vi "VI Server_GetControlClassNameAndType.vi"(7 "Label":string, 8 "error in (no error)":errorcluster, 11 "VI Server Cluster":T2) -> (0 "error out":errorcluster, 1 "ClassName":string, 2 "ControlType":T1, 3 "VI Server Cluster.DUP":T2)   [LabVIEW 2020, in "VI Server Toolkit LV2013.lvlib"]
doc: "Returns control class name and its type (digital, Boolean, etc.)\nRequires control's label input."
uses:
  VI Server Toolkit LV2013.lvlib
  VI Server_TypeDefs/VI Server_RefsCluster.ctl
  VI Server_TypeDefs/VI Server_DataType.ctl
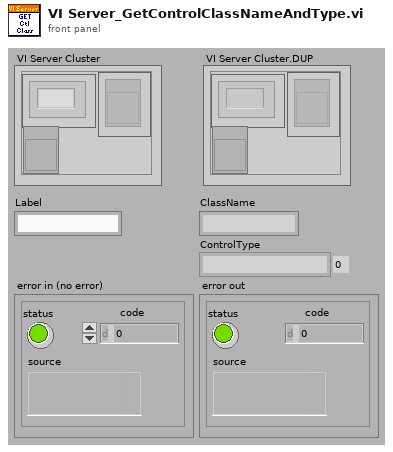
[diagram p1: front panel]
types:
  T1 = typedef "VI Server Toolkit LV2013.lvlib/VI Server_DataType.ctl" = enum16{"", "Digital [Dbl]", "Digital [Sgl]", "Digital [I32]", "Digital [I16]", "Digital [I8]", "Digital [U32]", "Digital [U16]", "Digital [U8]", "Boolean", "Slide [Dbl]", "Slide [Sgl]", "Slide [I32]", "Slide [I16]", "Slide [I8]", "Slide [U32]", "Slide [U16]", "Slide [U8]", "Enumerated", "Path", "VISA Resource Name", "Text Ring", "String", "TabControl", "Knob [U8]", "Knob [U16]", "Knob [U32]", "Knob [I8]", "Knob [I16]", "Knob [I32]", "Knob [SGL]", "Knob [DBL]"}
  T2 = typedef "VI Server_RefsCluster.ctl" = cluster{"Labels":string[], "Refs":refnum<vi>[], "VI Ref":refnum<vi>}
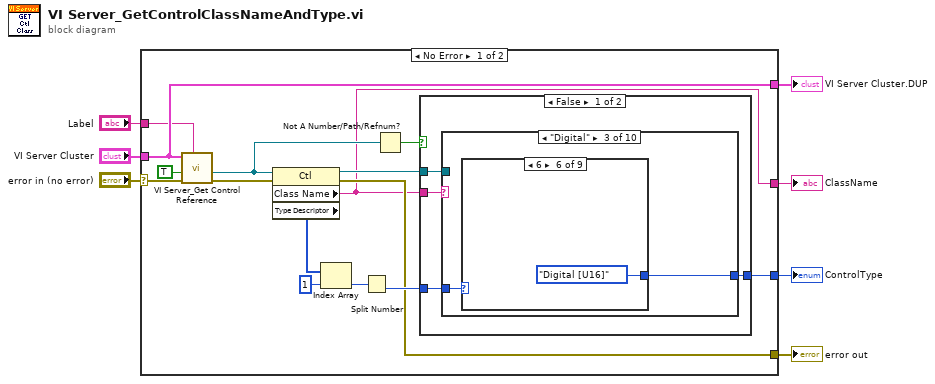
[diagram p0: block diagram]
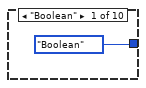
[diagram p2: hidden frame]
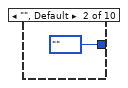
[diagram p3: hidden frame]
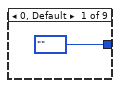
[diagram p4: hidden frame]
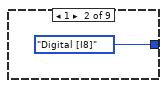
[diagram p5: hidden frame]
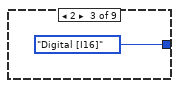
[diagram p6: hidden frame]
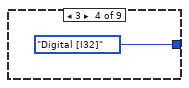
[diagram p7: hidden frame]
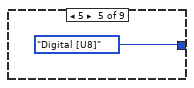
[diagram p8: hidden frame]
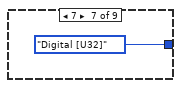
[diagram p9: hidden frame]
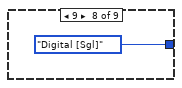
[diagram p10: hidden frame]
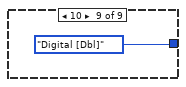
[diagram p11: hidden frame]
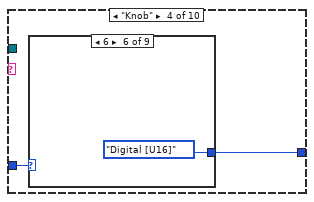
[diagram p12: hidden frame]
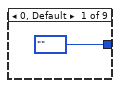
[diagram p13: hidden frame]
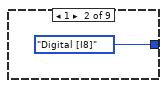
[diagram p14: hidden frame]
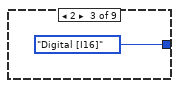
[diagram p15: hidden frame]
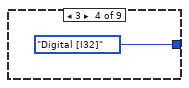
[diagram p16: hidden frame]
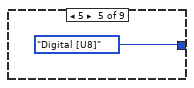
[diagram p17: hidden frame]
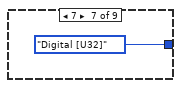
[diagram p18: hidden frame]
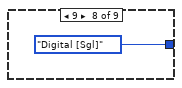
[diagram p19: hidden frame]
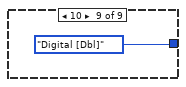
[diagram p20: hidden frame]
diagram:
  n1 = case shown="No Error" "error in (no error)" {
    selector: "error in (no error)" -> [w17 w69]
    tunnel: [w10 w69] -> w7
    tunnel: "VI Server Cluster" -> [w15 _]
    tunnel: "Label" -> [w14 _]
    tunnel: [w15 _] -> w3
    tunnel: [w11 VI_Server_DataType."" ("ControlType 2")] -> w2
    tunnel: [w9 _] -> w1
    frame No Error {
      n2 = call "VI Server_Get Control Reference.vi"("Label"=w14, "error in"=w17, "Single Instance (T)"=TRUE, "VI Server Cluster"=w15) -> ("error out"=w16:errorcluster, "Control Reference (Generic)"=w13:refnum<vi>)  [unwired: 4 in, 2 out]
      n3 = property class="Ctl"(reference=w13, error in=w16) -> (reference out=w18:refnum<vi>, error out=w10:errorcluster, "Class Name"=w9:string, "Type Descriptor"=w20:i16[])
      n4 = Index Array(array=w20, index=1) -> (element=w21:i16)
      n5 = Split Number(x=w21) -> (lo(x)=w19:u8)  [unwired: 1 out]
      n6 = Not A Number/Path/Refnum?(number/path/refnum=w13) -> (NaN/Path/Refnum?=w12:bool)
      n7 = case shown="False" w12 {
        tunnel: w9 -> [w26 _]
        tunnel: w19 -> [w25 _]
        tunnel: w18 -> [w24 _]
        tunnel: [w23 VI_Server_DataType."" ("ControlType 2")] -> w11
        frame False {
          n8 = case shown="\"Digital\"" w26 {
            tunnel: w25 -> [_ _ w30 w41 w52 _ _ _ _ _]
            tunnel: w24 -> [_ _ _ _ _ _ _ _ _ _]
            tunnel: [VI_Server_DataType."Boolean" ("ControlType 2") VI_Server_DataType."" ("ControlType 2") w29 w40 w51 VI_Server_DataType."Enumerated" ("ControlType 2") VI_Server_DataType."Path" ("ControlType 2") VI_Server_DataType."VISA Resource Name" ("ControlType 2") VI_Server_DataType."Text Ring" ("ControlType 2") VI_Server_DataType."String" ("ControlType 2")] -> w23
            frame "Boolean" {
            }
            frame "", Default {
            }
            frame "Digital" {
              n9 = case shown="6" w30 {
                tunnel: [VI_Server_DataType."" ("ControlType 2") VI_Server_DataType."Digital [I8]" ("ControlType 2") VI_Server_DataType."Digital [I16]" ("ControlType 2") VI_Server_DataType."Digital [I32]" ("ControlType 2") VI_Server_DataType."Digital [U8]" ("ControlType 2") VI_Server_DataType."Digital [U16]" ("ControlType 2") VI_Server_DataType."Digital [U32]" ("ControlType 2") VI_Server_DataType."Digital [Sgl]" ("ControlType 2") VI_Server_DataType."Digital [Dbl]" ("ControlType 2")] -> w29
                frame 0, Default {
                }
                frame 1 {
                }
                frame 2 {
                }
                frame 3 {
                }
                frame 5 {
                }
                frame 6 {
                }
                frame 7 {
                }
                frame 9 {
                }
                frame 10 {
                }
              }
            }
            frame "Knob" {
              n10 = case shown="6" w41 {
                tunnel: [VI_Server_DataType."" ("ControlType 2") VI_Server_DataType."Digital [I8]" ("ControlType 2") VI_Server_DataType."Digital [I16]" ("ControlType 2") VI_Server_DataType."Digital [I32]" ("ControlType 2") VI_Server_DataType."Digital [U8]" ("ControlType 2") VI_Server_DataType."Digital [U16]" ("ControlType 2") VI_Server_DataType."Digital [U32]" ("ControlType 2") VI_Server_DataType."Digital [Sgl]" ("ControlType 2") VI_Server_DataType."Digital [Dbl]" ("ControlType 2")] -> w40
                frame 0, Default {
                }
                frame 1 {
                }
                frame 2 {
                }
                frame 3 {
                }
                frame 5 {
                }
                frame 6 {
                }
                frame 7 {
                }
                frame 9 {
                }
                frame 10 {
                }
              }
            }
            frame "Slide" {
              n11 = case shown="0, Default" w52 {
                tunnel: [VI_Server_DataType."" ("ControlType 2") VI_Server_DataType."Digital [I8]" ("ControlType 2") VI_Server_DataType."Slide [I16]" ("ControlType 2") VI_Server_DataType."Slide [I32]" ("ControlType 2") VI_Server_DataType."Digital [U8]" ("ControlType 2") VI_Server_DataType."Digital [U16]" ("ControlType 2") VI_Server_DataType."Slide [U32]" ("ControlType 2") VI_Server_DataType."Slide [Sgl]" ("ControlType 2") VI_Server_DataType."Slide [Dbl]" ("ControlType 2")] -> w51
                frame 0, Default {
                }
                frame 1 {
                }
                frame 2 {
                }
                frame 3 {
                }
                frame 5 {
                }
                frame 6 {
                }
                frame 7 {
                }
                frame 9 {
                }
                frame 10 {
                }
              }
            }
            frame "Enum" {
            }
            frame "Path" {
            }
            frame "VISAResourceName" {
            }
            frame "Ring" {
            }
            frame "String" {
            }
          }
        }
        frame True {
          (unwired) ""
        }
      }
    }
    frame Error {
    }
  }
  "error out" <- w7
  "VI Server Cluster.DUP" <- w3
  "ControlType" <- w2
  "ClassName" <- w1
